vi "Slider_Recorder.vi"(7 "Slider":dbl(slide) scale=0.0..10.0, 11 "Error_In":errorcluster) -> (15 "Error_Out":errorcluster)   [LabVIEW 2021]
doc: "This is the main module to generate the data ( Recording the data )"
uses:
  Controls/Operation.ctl
  LV2/UE_C_LV2.vi
  Controls/Event_Data.ctl
  Controls/Event_Data_and_Parameter.ctl
panel:
  out "Record_State":string
  in  "PlayBack?":bool
  # "Note: Press the slider to start recording. Release the slider to stop recording."
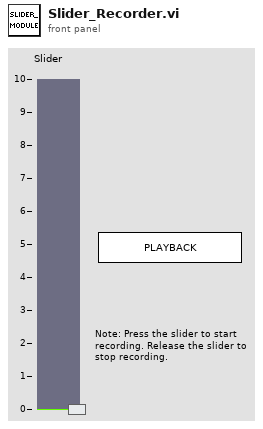
[diagram p1: front panel]
types:
  T1 = enum8{"Enabled", "Disabled", "Disabled and Grayed Out"}
  T2 = typedef "Event_Data.ctl" = cluster{"Event_Data":dbl, "PlayBack?":bool}
  T3 = typedef "Event_Data_and_Parameter.ctl" = cluster{"Event_Data":dbl[], "Generate_Event":bool, "Playback?":bool, "Index":i32}
  T4 = typedef "Operation.ctl" = enum16{"Create_UE", "Generate_UE", "Destroy_UE", "Get_UE_Reference"}
  T5 = enum32{"Bad", "Idle", "Run top level", "Running"}
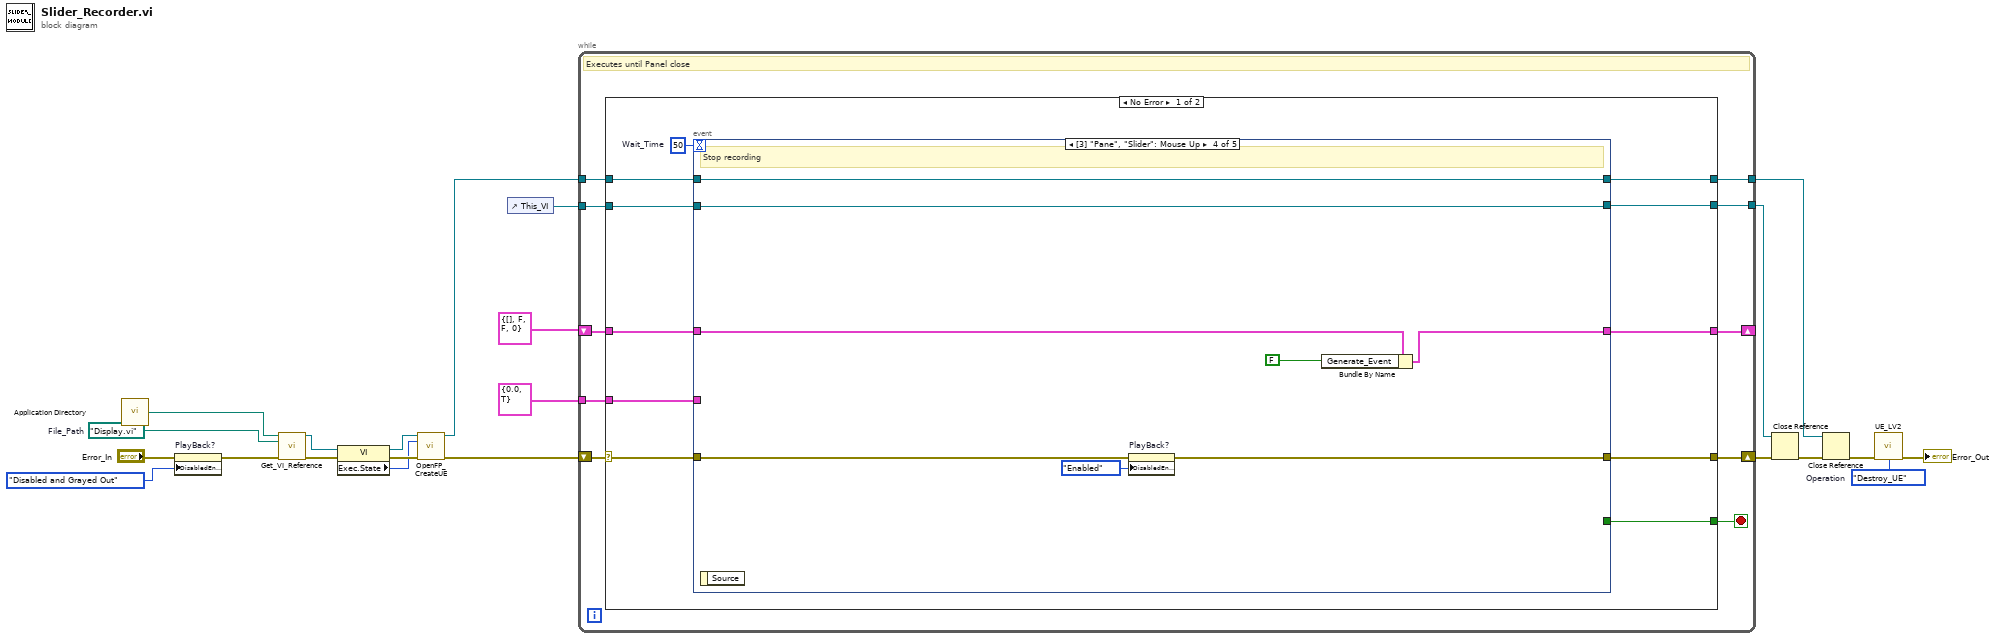
[diagram p0: block diagram]
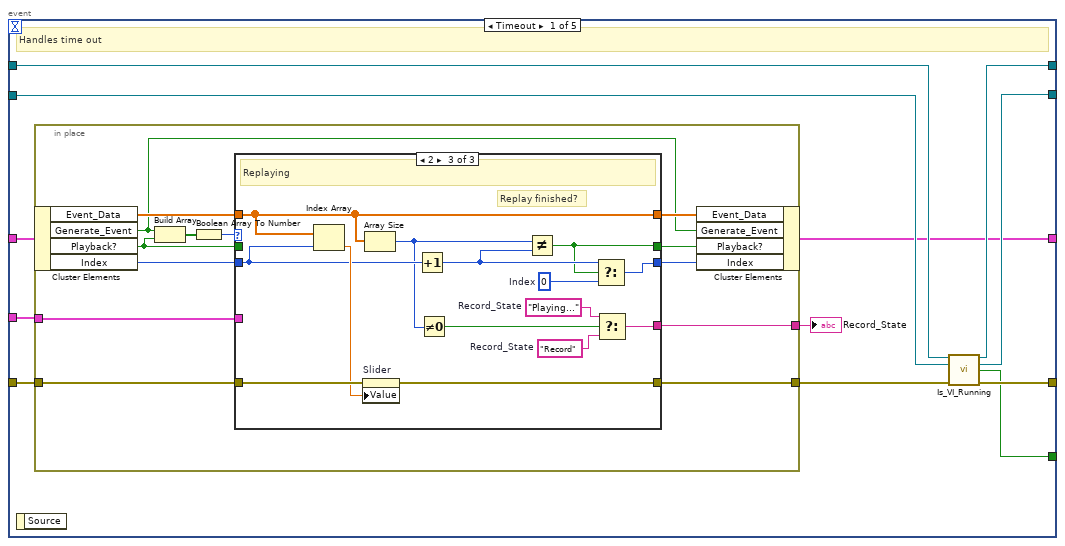
[diagram p2: hidden frame]
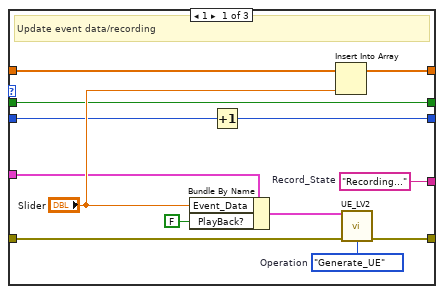
[diagram p3: hidden frame]
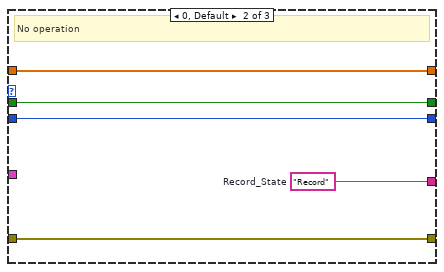
[diagram p4: hidden frame]
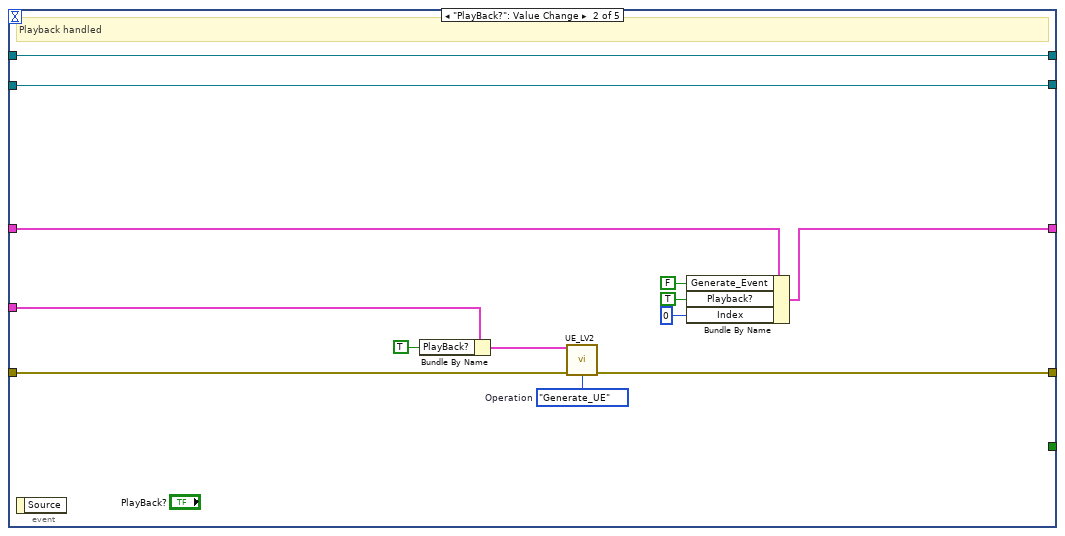
[diagram p5: hidden frame]
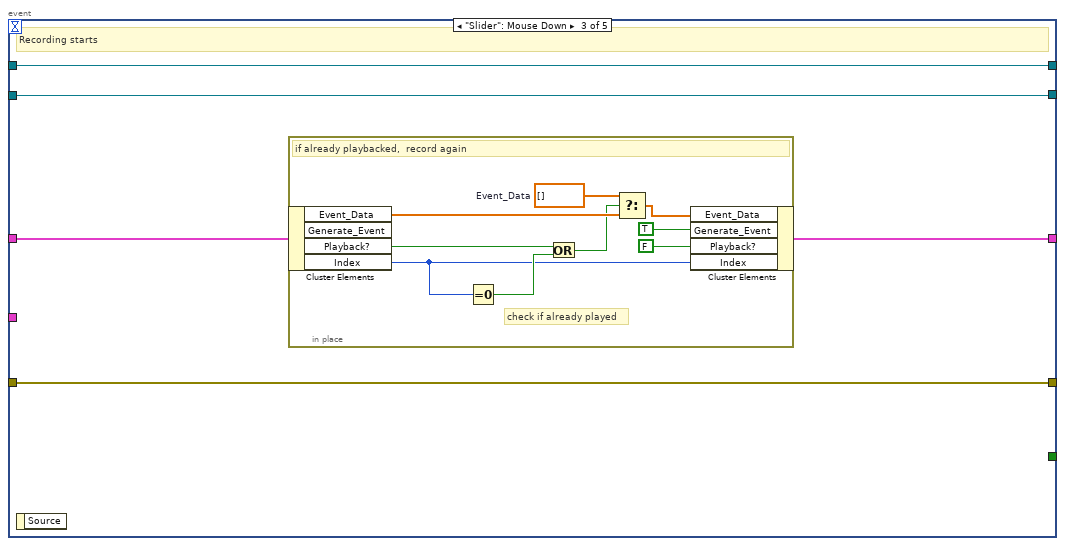
[diagram p6: hidden frame]
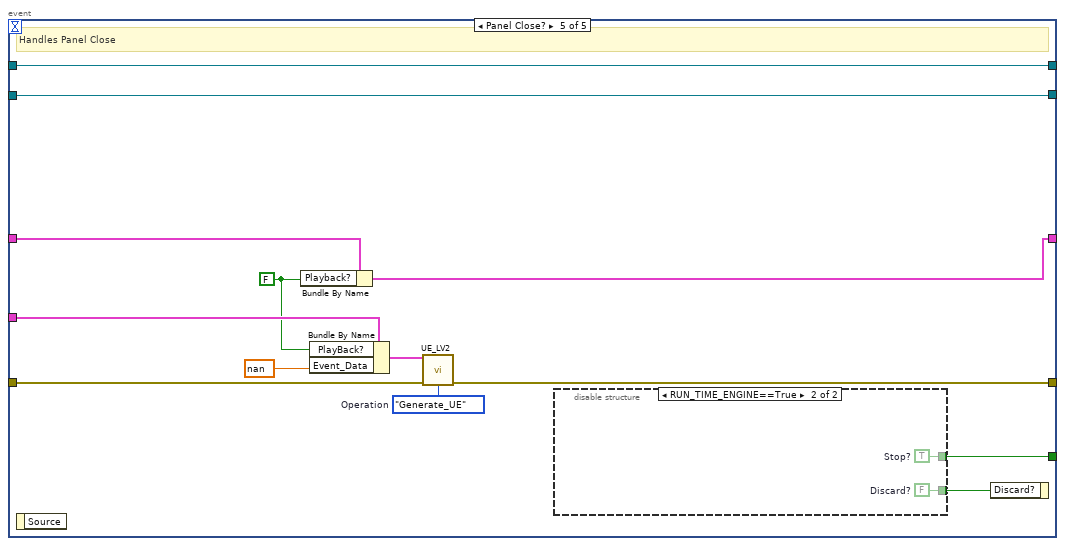
[diagram p7: hidden frame]
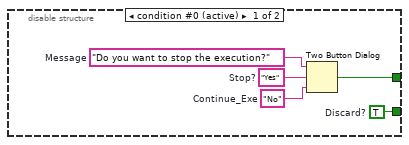
[diagram p8: hidden frame]
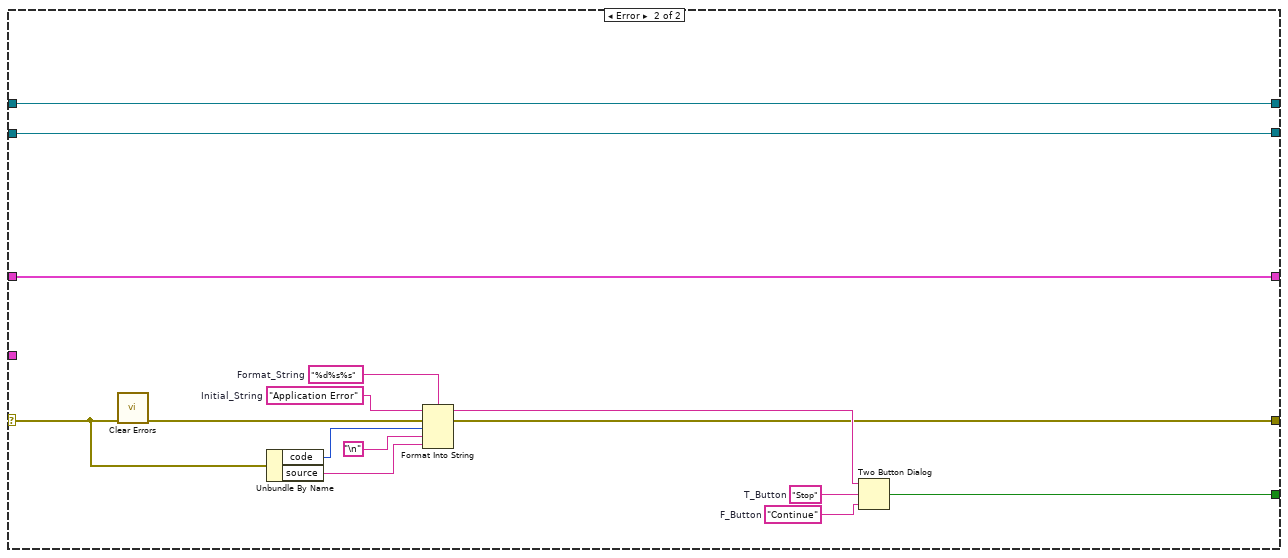
[diagram p9: hidden frame]
diagram:
  w16 = Operation."Destroy_UE"  # Operation
  w20 = path "Display.vi"  # File_Path
  n1 = call <vilib>:"Application Directory.vi"() -> ("Application Directory"=w21:path)
  n2 = property on="PlayBack?" class="Bool"(error in="Error_In", "DisabledEnum"=T1."Disabled and Grayed Out" ("Disabled")) -> (error out=w2:errorcluster)  [unwired: 1 in, 1 out]
  n3 = call "Get_VI_Reference.vi"("Application_Directory"=w21, "File_Path"=w20, "Error_In"=w2) -> ("VI_Reference"=w19:refnum<vi>, "Error_Out"=w22:errorcluster)  [unwired: 11 in]
  n4 = property on="Property Node" class="VI"(reference=w19, error in=w22) -> (reference out=w8:refnum<vi>, error out=w9:errorcluster, "Exec.State"=w7:T5)
  n5 = call "OpenFP_CreateUE.vi"("VI_Reference_In"=w8, "Exec.State"=w7, "Error_In"=w9) -> ("VI_Reference_Out"=w6:refnum<vi>, "Error_Out"=w3:errorcluster)  [unwired: 11 in]
  n6 = control-ref of="This_VI"() -> (w15:refnum<vi>)
  n7 = while {
    shift-right: [w29] -> _
    shift-left: T3 {"Event_Data"=[], "Generate_Event"=FALSE, "Playback?"=FALSE, "Index"=0} -> [w28]
    tunnel: w6 -> [w27]
    tunnel: w15 -> [w26]
    tunnel: [w25] -> w14
    tunnel: [w24] -> w11
    tunnel: T2 {"Event_Data"=0.0, "PlayBack?"=TRUE} ("Event_Data") -> [w23]
    shift-right: [w31] -> w18
    shift-left: w3 -> [w32]
    stop <- w30 stop-if-true
    # "Executes until Panel close"
    n8 = case shown="No Error" w32 {
      selector: w32 -> [w42 w162]
      tunnel: [w43 w163] -> w31
      tunnel: [w40 w159] -> w30
      tunnel: [w34 w158] -> w29
      tunnel: w28 -> [w39 w158]
      tunnel: w27 -> [w38 w157]
      tunnel: w26 -> [w37 w156]
      tunnel: [w36 w156] -> w25
      tunnel: [w35 w157] -> w24
      tunnel: w23 -> [w33 _]
      frame No Error {
        w41 = 50  # Wait_Time
        n9 = event shown="[3] \"Pane\", \"Slider\": Mouse Up" {
          selector: _ -> [_ _ _ _ _]
          dyn-events: _ -> [_ _ _ _ _]
          timeout: w41 -> [_ _ _ _ _]
          tunnel: [w53 w112 w118 w129 w140] -> w43
          tunnel: w42 -> [w55 w113 w118 w134 w146]
          tunnel: [w48 _ _ _ w137] -> w40
          tunnel: w39 -> [w47 w108 w115 w135 w143]
          tunnel: w38 -> [w52 w102 w117 w131 w147]
          tunnel: w37 -> [w51 w103 w116 w130 w148]
          tunnel: [w50 w103 w116 w130 w148] -> w36
          tunnel: [w49 w102 w117 w131 w147] -> w35
          tunnel: [w46 w107 w114 w133 w142] -> w34
          tunnel: w33 -> [w44 w101 _ _ w141]
          event Timeout {
            # "Handles time out"
            n10 = event-data() -> ()  [unwired: 1 in, 1 out]
            n11 = in-place "In Place Element Structure" {
              in-place-border: w55 -> [w68]
              in-place-border: [w65] -> w54
              in-place-border: [w60] -> w45
              in-place-border: w44 -> [w59]
              n12 = in-place-cluster #1(w47) -> ("Event_Data"=w64:dbl[], "Generate_Event"=w61:bool, "Playback?"=w57:bool, "Index"=w56:i32)
              n13 = Build Array(w61, w57) -> (w67:bool[])
              n14 = Boolean Array To Number(Boolean array=w67) -> (number=w66:u32)
              n15 = case shown="2" w66 {
                tunnel: w68 -> [w81 w84 w100]
                tunnel: [w80 w84 w99] -> w65
                tunnel: [w78 w86 w97] -> w63
                tunnel: w64 -> [w77 w86 w97]
                tunnel: [w69 w85 w96] -> w62
                tunnel: w56 -> [w70 w85 w90]
                tunnel: [w73 w82 w92] -> w60
                tunnel: w59 -> [w72 _ _]
                tunnel: [w71 w83 w89] -> w58
                tunnel: w57 -> [w71 w83 _]
                frame 1 {
                  w73 = "Recording..."  # Record_State
                  w79 = Operation."Generate_UE"  # Operation
                  # "Update event data/recording"
                  n16 = Bundle By Name(cluster=w72, "Event_Data"="Slider", "PlayBack?"=FALSE) -> (w75:T2)
                  n17 = Increment(x=w70) -> (x+1=w69:i32)
                  n18 = Insert Into Array(array=w77, new element="Slider") -> (w78:dbl[])  [unwired: 1 in]
                  n19 = call-poly "UE_LV2.vi"("Event_Data"=w75, "Error_In"=w81, "Operation"=w79) -> ("Error_Out"=w80:errorcluster)  [unwired: 11 in, 1 out]
                }
                frame 0, Default {
                  w82 = "Record"  # Record_State
                  # "No operation"
                }
                frame 2 {
                  w91 = "Record"  # Record_State
                  w95 = 0  # Index
                  w93 = "Playing..."  # Record_State
                  # "Replay finished?"
                  # "Replaying"
                  n20 = Index Array(array=w97, index=w90) -> (element=w98:dbl)
                  n21 = property on="Slider" class="Slide (strict)"(error in=w100, "Value"=w98) -> (error out=w99:errorcluster)  [unwired: 1 in, 1 out]
                  n22 = Array Size(array=w97) -> (size(s)=w88:i32)
                  n23 = Increment(x=w90) -> (x+1=w94:i32)
                  n24 = Not Equal To 0?(x=w88) -> (x != 0?=w87:bool)
                  n25 = Not Equal?(x=w88, y=w94) -> (x != y?=w89:bool)
                  n26 = Select(t=w94, s=w89, f=w95) -> (s? t:f=w96:i32)
                  n27 = Select(t=w93, s=w87, f=w91) -> (s? t:f=w92:string)
                }
              }
              n28 = in-place-cluster #1("Event_Data"=w63, "Generate_Event"=w61, "Playback?"=w58, "Index"=w62) -> (w46:T3)
            }
            "Record_State" <- w45
            n29 = call "Is_VI_Running.vi"("Other_VI_Reference_In"=w52, "This_VI_Reference_In"=w51, "Error_In"=w54) -> ("Other_VI_Reference_Out"=w49:refnum<vi>, "This_VI_Reference_Out"=w50:refnum<vi>, "Stop"=w48:bool, "Error_Out"=w53:errorcluster)  [unwired: 9 in]
          }
          event "PlayBack?": Value Change {
            w111 = Operation."Generate_UE"  # Operation
            # "Playback handled"
            n30 = event-data() -> ()  [unwired: 1 in, 1 out]
            n31 = Bundle By Name(cluster=w101, "PlayBack?"=TRUE) -> (w110:T2)
            n32 = call-poly "UE_LV2.vi"("Event_Data"=w110, "Error_In"=w113, "Operation"=w111) -> ("Error_Out"=w112:errorcluster)  [unwired: 11 in, 1 out]
            n33 = Bundle By Name(cluster=w108, "Generate_Event"=FALSE, "Playback?"=TRUE, "Index"=0) -> (w107:T3)
          }
          event "Slider": Mouse Down {
            # "Recording starts"
            n34 = event-data() -> ()  [unwired: 1 in, 1 out]
            n35 = in-place "In Place Element Structure" {
              w124 = dbl[] []  # Event_Data
              # "check if already played"
              # "if already playbacked,  record again"
              n36 = in-place-cluster #2(w115) -> ("Event_Data"=w123:dbl[], "Playback?"=w119:bool, "Index"=w121:i32)  [unwired: 1 out]
              n37 = Equal To 0?(x=w121) -> (x = 0?=w122:bool)
              n38 = Or(x=w119, y=w122) -> (x .or. y?=w120:bool)
              n39 = Select(t=w124, s=w120, f=w123) -> (s? t:f=w125:dbl[])
              n40 = in-place-cluster #2("Event_Data"=w125, "Generate_Event"=TRUE, "Playback?"=FALSE, "Index"=w121) -> (w114:T3)
            }
          }
          event "Slider": Mouse Up {
            # "Stop recording"
            n41 = event-data() -> ()  [unwired: 1 in, 1 out]
            n42 = property on="PlayBack?" class="Bool"(error in=w134, "DisabledEnum"=T1."Enabled" ("Disabled")) -> (error out=w129:errorcluster)  [unwired: 1 in, 1 out]
            n43 = Bundle By Name(cluster=w135, "Generate_Event"=FALSE) -> (w133:T3)
          }
          event Panel Close? {
            w138 = FALSE
            w145 = Operation."Generate_UE"  # Operation
            # "Handles Panel Close"
            n44 = event-data() -> ()  [unwired: 1 in, 1 out]
            n45 = Bundle By Name(cluster=w143, "Playback?"=w138) -> (w142:T3)
            n46 = Bundle By Name(cluster=w141, "PlayBack?"=w138, "Event_Data"=nan) -> (w144:T2)
            n47 = call-poly "UE_LV2.vi"("Event_Data"=w144, "Error_In"=w146, "Operation"=w145) -> ("Error_Out"=w140:errorcluster)  [unwired: 11 in, 1 out]
            n48 = disable-structure shown="RUN_TIME_ENGINE==True" {
              disable-tunnel: [w150 w155] -> w137
              disable-tunnel: [w149 w154] -> w136
              frame condition #0 (active) {
                w149 = TRUE  # Discard?
                w151 = "No"  # Continue_Exe
                w152 = "Yes"  # Stop?
                w153 = "Do you want to stop the execution?"  # Message
                n49 = Two Button Dialog(message=w153, 1:w151, 2:w152) -> (T button?=w150:bool)
              }
              frame condition #1 {
                w154 = FALSE  # Discard?
                w155 = TRUE  # Stop?
              }
            }
            n50 = event-data ("Event Filter Node")("Discard?"=w136) -> ()  [unwired: 1 in, 1 out]
          }
        }
      }
      frame Error {
        w166 = "%d%s%s"  # Format_String
        w167 = "Application Error"  # Initial_String
        w168 = "Stop"  # T_Button
        w169 = "Continue"  # F_Button
        n51 = call <vilib>:"Clear Errors.vi"("error in (no error)"=w162) -> ("error out"=w164:errorcluster)  [unwired: 5 in, 1 out]
        n52 = Unbundle By Name(w162) -> ("code"=w161:i32, "source"=w160:string)
        n53 = Format Into String(format string=w166, initial string=w167, error in=w164, w161, "\n" ("Line Feed Constant"), w160) -> (resulting string=w170:string, error out=w163:errorcluster)
        n54 = Two Button Dialog(message=w170, 1:w169, 2:w168) -> (T button?=w159:bool)
      }
    }
  }
  n55 = Close Reference(reference=w14, error in (no error)=w18) -> (error out=w13:errorcluster)
  n56 = Close Reference(reference=w11, error in (no error)=w13) -> (error out=w12:errorcluster)
  n57 = call-poly "UE_LV2.vi"("Error_In"=w12, "Operation"=w16) -> ("Error_Out"=→"Error_Out":errorcluster)  [unwired: 12 in, 1 out]
